vi "MoveGOSSIP_out.vi"(8 "error in (no error)":errorcluster) -> (0 "error out":errorcluster, 3 "In range is True":bool)   [LabVIEW 2020]
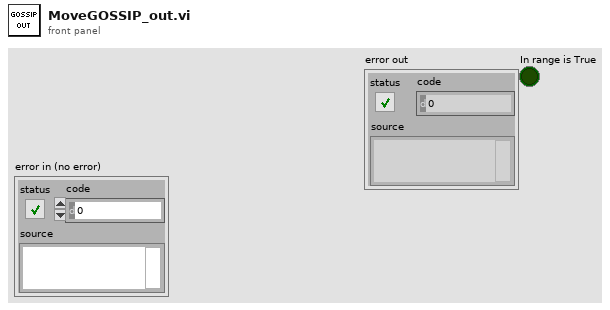
[diagram p1: front panel]
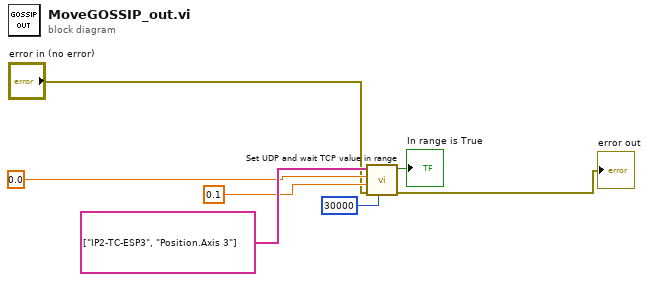
[diagram p0: block diagram]
diagram:
  n1 = call "Set UDP and wait TCP value in range.vi"("timeout"=u32 30000, "error in (no error)"="error in (no error)", "tolerance"=0.1, "set value"=0.0, "device and variable"=string[] ["IP2-TC-ESP3", "Position.Axis 3"]) -> ("error out"=→"error out":errorcluster, "In range is True"=→"In range is True":bool)  [unwired: 5 in]
